vi "Block DMA.vi"() -> ()   [LabVIEW 2016]
uses:
  <vilib>/NI/GE Reflective Memory Driver/Typedefs/GE 5565PIORC.Typedef.DMA Wait Mode.ctl
  <vilib>/NI/GE Reflective Memory Driver/GE 5565PIORC.lvclass/GE 5565PIORC.ctl
  <vilib>/NI/GE Reflective Memory Driver/Methods/GE 5565PIORC.DMA.Block.Write (String).vi
  <vilib>/NI/GE Reflective Memory Driver/Methods/GE 5565PIORC.DMA.Create Transfer (Block).vi
  <vilib>/NI/GE Reflective Memory Driver/Methods/GE 5565PIORC.DMA.Get Transfer Components (Block).vi
  <vilib>/NI/GE Reflective Memory Driver/Methods/GE 5565PIORC.DMA.Block.Read (String).vi
  <vilib>/NI/GE Reflective Memory Driver/Properties/Registers/GE 5565PIORC.Registers.LAS1RR.PCI Address Range.Get.vi
  <vilib>/NI/GE Reflective Memory Driver/Methods/GE 5565PIORC.PXI Interrupts.Enable.vi
  <vilib>/NI/GE Reflective Memory Driver/Properties/Registers/GE 5565PIORC.Registers.DMACSR0.Channel 0 Enable.Set.vi
  <vilib>/NI/GE Reflective Memory Driver/Properties/Registers/GE 5565PIORC.Registers.INTCSR.Local DMA Channel 0 Interrupt Enable.Set.vi
  <vilib>/NI/GE Reflective Memory Driver/Properties/GE 5565PIORC.Read VISA MEMACC.vi
  <vilib>/NI/GE Reflective Memory Driver/Methods/GE 5565PIORC.DMA.Create Transfer (Scatter-Gather).vi
  <vilib>/NI/GE Reflective Memory Driver/Methods/GE 5565PIORC.DMA.Configure.vi
  <vilib>/NI/GE Reflective Memory Driver/Methods/GE 5565PIORC.PXI Interrupts.Discard Events.vi
  <vilib>/NI/GE Reflective Memory Driver/Methods/GE 5565PIORC.DMA.Start.vi
  <vilib>/NI/GE Reflective Memory Driver/Methods/GE 5565PIORC.DMA.Wait for Done.vi
  <vilib>/NI/GE Reflective Memory Driver/Methods/GE 5565PIORC.DMA.Block.Clear.vi
  <vilib>/NI/GE Reflective Memory Driver/Methods/GE 5565PIORC.DMA.Block.Clear (multiple).vi
  <vilib>/NI/GE Reflective Memory Driver/Properties/Registers/GE 5565PIORC.Registers.Local Configuration.Read.vi
  <vilib>/NI/GE Reflective Memory Driver/Properties/Registers/GE 5565PIORC.Registers.Local Configuration.Read (U32).vi
  <vilib>/NI/GE Reflective Memory Driver/Properties/Registers/GE 5565PIORC.Registers.Local Configuration.Read (U8).vi
  <vilib>/NI/GE Reflective Memory Driver/Properties/Registers/GE 5565PIORC.Registers.Local Configuration.Write.vi
  <vilib>/NI/GE Reflective Memory Driver/Properties/Registers/GE 5565PIORC.Registers.Local Configuration.Write (U8).vi
  <vilib>/NI/GE Reflective Memory Driver/Methods/GE 5565PIORC.Bit Manipulation.Set Bit.vi
  <vilib>/NI/GE Reflective Memory Driver/Methods/GE 5565PIORC.Bit Manipulation.Set Bit (U8).vi
  <vilib>/NI/GE Reflective Memory Driver/Properties/Registers/GE 5565PIORC.Registers.Local Configuration.Write (U32).vi
  <vilib>/NI/GE Reflective Memory Driver/Methods/GE 5565PIORC.Bit Manipulation.Set Bit (U32).vi
  <vilib>/NI/GE Reflective Memory Driver/Methods/GE 5565PIORC.DMA.Size.vi
  <vilib>/NI/GE Reflective Memory Driver/Properties/Registers/GE 5565PIORC.Registers.DMADPR0.Direction of Transfer.Set.vi
  <vilib>/NI/GE Reflective Memory Driver/Properties/Registers/GE 5565PIORC.Registers.DMASIZ0.DMA Transfer Size.Set.vi
  <vilib>/NI/GE Reflective Memory Driver/Properties/Registers/GE 5565PIORC.Registers.DMALADR0.Local Address Register.Set.vi
  <vilib>/NI/GE Reflective Memory Driver/Properties/Registers/GE 5565PIORC.Registers.DMAMODE0.Scatter-Gather Mode.Set.vi
  <vilib>/NI/GE Reflective Memory Driver/Properties/Registers/GE 5565PIORC.Registers.DMAPADR0.PCI Address Register.Set.vi
  <vilib>/NI/GE Reflective Memory Driver/Methods/GE 5565PIORC.DMA.Scatter-Gather.Link Block Descriptors.vi
  <vilib>/NI/GE Reflective Memory Driver/Methods/GE 5565PIORC.DMA.Scatter-Gather.Commit Linked Block Descriptors.vi
  <vilib>/NI/GE Reflective Memory Driver/Properties/Registers/GE 5565PIORC.Registers.DMADPR0.Channel 0 First Descriptor Address.Set.vi
  <vilib>/NI/GE Reflective Memory Driver/Methods/GE 5565PIORC.DMA.Get Transfer Components (Scatter-Gather).vi
  <vilib>/Utility/error.llb/Clear Errors.vi
  <vilib>/NI/GE Reflective Memory Driver/Properties/Registers/GE 5565PIORC.Registers.DMACSR0.Channel 0 Start.Set.vi
  <vilib>/NI/GE Reflective Memory Driver/Properties/Registers/GE 5565PIORC.Registers.DMACSR0.Channel 0 Clear Interrupt.Set.vi
  <vilib>/NI/GE Reflective Memory Driver/Methods/GE 5565PIORC.DMA.Poll for Done Signal.vi
  <vilib>/NI/GE Reflective Memory Driver/Methods/GE 5565PIORC.PXI Interrupts.Wait for Event.vi
  <vilib>/NI/GE Reflective Memory Driver/Methods/GE 5565PIORC.DMA.Block.Clear (single).vi
  <vilib>/NI/GE Reflective Memory Driver/Methods/GE 5565PIORC.Registers.Read.vi
  <vilib>/NI/GE Reflective Memory Driver/Methods/GE 5565PIORC.Registers.Read (U32).vi
  <vilib>/NI/GE Reflective Memory Driver/Methods/GE 5565PIORC.Registers.Read (U8).vi
  <vilib>/NI/GE Reflective Memory Driver/Methods/GE 5565PIORC.Registers.Write.vi
  <vilib>/NI/GE Reflective Memory Driver/Methods/GE 5565PIORC.Registers.Write (U8).vi
  <vilib>/NI/GE Reflective Memory Driver/Methods/GE 5565PIORC.Registers.Write (U32).vi
  <vilib>/NI/GE Reflective Memory Driver/Methods/GE 5565PIORC.DMA.Scatter-Gather.Set Descriptor Params.vi
  <vilib>/NI/GE Reflective Memory Driver/Methods/GE 5565PIORC.DMA.Is Done.vi
  <vilib>/NI/GE Reflective Memory Driver/Properties/Registers/GE 5565PIORC.Registers.DMACSR0.Channel 0 Inactive.Get.vi
  <vilib>/NI/GE Reflective Memory Driver/Methods/GE 5565PIORC.Bit Manipulation.Get Bit.vi
  <vilib>/NI/GE Reflective Memory Driver/Methods/GE 5565PIORC.Bit Manipulation.Get Bit (U8).vi
  <vilib>/NI/GE Reflective Memory Driver/Methods/GE 5565PIORC.Round Up to Nearest 8.vi
  <vilib>/NI/GE Reflective Memory Driver/Methods/GE 5565PIORC.Round Up to Nearest 16.vi
  <vilib>/NI/GE Reflective Memory Driver/GE 5565PIORC.lvclass
panel:
  out "Success?":bool
  out "Read Timed Out?":bool
  out "Write Timed Out?":bool
  in  "RFM offset":u32 format="%.0x"
  in  "Transfer Size (bytes)":u32=1024000
  in  "Wait Mode":T1
  in  "VISA Resource Name":refnum<visa-resource-name>="PXI4::14::INSTR"
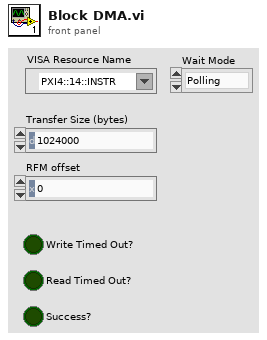
[diagram p1: front panel]
types:
  T1 = typedef "GE 5565PIORC.lvclass/GE 5565PIORC.Typedef.DMA Wait Mode.ctl" = enum16{"Polling", "Interrupt"}
  T2 = typedef "GE 5565PIORC.lvclass/GE 5565PIORC.Typedef.DMA Block Descriptor.ctl" = cluster{"descriptor ptr (VISA)":u32, "descriptor ptr (RFM)":u32, "descriptor size":u32, "descriptor params":T3}
  T3 = typedef "GE 5565PIORC.lvclass/GE 5565PIORC.Typedef.DMA Block Descriptor Params.ctl" = cluster{"data ptr (lower)":u32, "data ptr (upper)":u32, "data size":u32, "next descriptor ptr":u32}
  T4 = typedef "GE 5565PIORC.lvclass/GE 5565PIORC.Typedef.DMA Transfer Spec.ctl" = cluster{"RFM offset":u32, "Block Descriptors":T2[]}
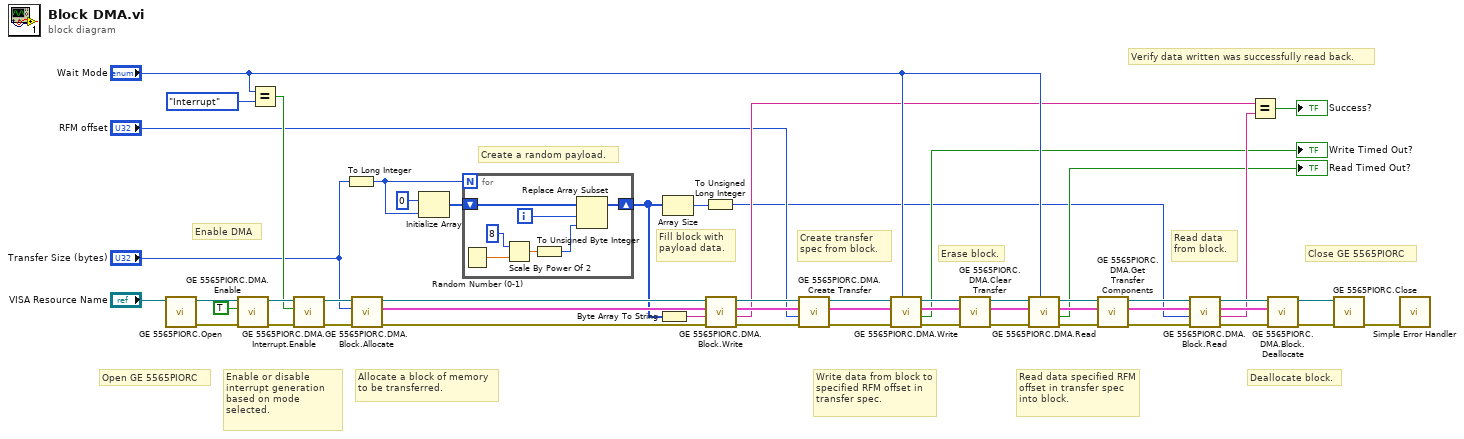
[diagram p0: block diagram]
diagram:
  # "Verify data written was successfully read back."
  # "Close GE 5565PIORC"
  # "Deallocate block."
  # "Erase block."
  # "Read data from block."
  # "Read data specified RFM offset in transfer spec into block."
  # "Write data from block to specified RFM offset in transfer spec."
  # "Create transfer spec from block."
  # "Fill block with payload data."
  # "Allocate a block of memory to be transferred."
  # "Enable or disable interrupt generation based on mode selected."
  # "Enable DMA"
  # "Open GE 5565PIORC"
  # "Create a random payload."
  n1 = call <vilib>:"GE 5565PIORC.Open.vi"("VISA resource name"="VISA Resource Name") -> ("error out"=w50:errorcluster, "GE 5565PIORC"=w51:refnum<class "GE 5565PIORC.lvclass">)  [unwired: 9 in]
  n2 = call <vilib>:"GE 5565PIORC.DMA.Enable.vi"("error in (no error)"=w50, "enable (T)"=TRUE, "GE 5565PIORC in"=w51) -> ("error out"=w48:errorcluster, "GE 5565PIORC out"=w47:refnum<class "GE 5565PIORC.lvclass">)  [unwired: 7 in]
  n3 = Equal?(x="Wait Mode", y=GE_5565PIORC.Typedef.DMA_Wait_Mode."Interrupt") -> (x = y?=w38:bool)
  n4 = call <vilib>:"GE 5565PIORC.DMA.Interrupt.Enable.vi"("error in (no error)"=w48, "enable (T)"=w38, "GE 5565PIORC in"=w47) -> ("error out"=w44:errorcluster, "GE 5565PIORC out"=w45:refnum<class "GE 5565PIORC.lvclass">)  [unwired: 7 in]
  n5 = To Long Integer(number="Transfer Size (bytes)") -> (32bit integer=w32:i32)
  n6 = call <vilib>:"GE 5565PIORC.DMA.Block.Allocate.vi"("error in (no error)"=w44, "size in bytes"="Transfer Size (bytes)", "GE 5565PIORC in"=w45) -> ("error out"=w25:errorcluster, "Block Descriptor"=w22:T2, "GE 5565PIORC out"=w26:refnum<class "GE 5565PIORC.lvclass">)  [unwired: 6 in]
  n7 = Initialize Array(u8 0, w32) -> (w42:u8[])
  n8 = for {
    N: w32 -> [_]
    shift-right: [w58] -> w18
    shift-left: w42 -> [w59]
    i -> [w57]
    n9 = Random Number (0-1)() -> (number: 0 to 1=w56:dbl)
    n10 = Scale By Power Of 2(n=i16 8, x=w56) -> (x*2^n=w54:dbl)
    n11 = To Unsigned Byte Integer(number=w54) -> (unsigned 8bit integer=w53:u8)
    n12 = Replace Array Subset(array=w59, new element=w53, index=w57) -> (w58:u8[])
  }
  n13 = Byte Array To String(unsigned byte array=w18) -> (string=w19:string)
  n14 = Array Size(array=w18) -> (size(s)=w4:i32)
  n15 = To Unsigned Long Integer(number=w4) -> (unsigned 32bit integer=w1:u32)
  n16 = call-poly <vilib>:"GE 5565PIORC.DMA.Block.Write.vi"("error in (no error)"=w25, "data"=w19, "Block Descriptor in"=w22, "GE 5565PIORC in"=w26) -> ("error out"=w23:errorcluster, "data out"=w20:string, "Block Descriptor out"=w21:T2, "GE 5565PIORC out"=w24:refnum<class "GE 5565PIORC.lvclass">)  [unwired: 4 in]
  n17 = call-poly <vilib>:"GE 5565PIORC.DMA.Create Transfer.vi"("error in (no error)"=w23, "RFM offset"="RFM offset", "Block Descriptor"=w21, "GE 5565PIORC in"=w24) -> ("error out"=w39:errorcluster, "DMA Transfer Spec"=w40:T4, "GE 5565PIORC out"=w41:refnum<class "GE 5565PIORC.lvclass">)  [unwired: 4 in, 1 out]
  n18 = call <vilib>:"GE 5565PIORC.DMA.Write.vi"("wait mode (polling)"="Wait Mode", "error in (no error)"=w39, "DMA Transfer Spec"=w40, "GE 5565PIORC in"=w41) -> ("error out"=w16:errorcluster, "timed out?"=→"Write Timed Out?":bool, "DMA Transfer Spec dup"=w15:T4, "GE 5565PIORC out"=w17:refnum<class "GE 5565PIORC.lvclass">)  [unwired: 4 in]
  n19 = call <vilib>:"GE 5565PIORC.DMA.Clear Transfer.vi"("error in (no error)"=w16, "DMA Transfer Spec in"=w15, "GE 5565PIORC in"=w17) -> ("error out"=w13:errorcluster, "DMA Transfer Spec out"=w12:T4, "GE 5565PIORC out"=w14:refnum<class "GE 5565PIORC.lvclass">)  [unwired: 6 in]
  n20 = call <vilib>:"GE 5565PIORC.DMA.Read.vi"("wait mode (polling)"="Wait Mode", "error in (no error)"=w13, "DMA Transfer Spec"=w12, "GE 5565PIORC in"=w14) -> ("error out"=w9:errorcluster, "timed out?"=→"Read Timed Out?":bool, "DMA Transfer Spec dup"=w8:T4, "GE 5565PIORC out"=w10:refnum<class "GE 5565PIORC.lvclass">)  [unwired: 4 in]
  n21 = call-poly <vilib>:"GE 5565PIORC.DMA.Get Transfer Components.vi"("error in (no error)"=w9, "DMA Transfer Spec in"=w8, "GE 5565PIORC in"=w10) -> ("error out"=w5:errorcluster, "Block Descriptor"=w6:T2, "GE 5565PIORC out"=w7:refnum<class "GE 5565PIORC.lvclass">)  [unwired: 5 in, 1 out]
  n22 = call-poly <vilib>:"GE 5565PIORC.DMA.Block.Read.vi"("error in (no error)"=w5, "bytes to read"=w1, "Block Descriptor in"=w6, "GE 5565PIORC in"=w7) -> ("error out"=w29:errorcluster, "data"=w27:string, "Block Descriptor out"=w28:T2, "GE 5565PIORC out"=w30:refnum<class "GE 5565PIORC.lvclass">)  [unwired: 4 in]
  n23 = Equal?(x=w20, y=w27) -> (x = y?=→"Success?":bool)
  n24 = call <vilib>:"GE 5565PIORC.DMA.Block.Deallocate.vi"("error in (no error)"=w29, "Block Descriptor"=w28, "GE 5565PIORC in"=w30) -> ("error out"=w35:errorcluster, "GE 5565PIORC out"=w36:refnum<class "GE 5565PIORC.lvclass">)  [unwired: 7 in]
  n25 = call <vilib>:"GE 5565PIORC.Close.vi"("error in (no error)"=w35, "GE 5565PIORC in"=w36) -> ("error out"=w34:errorcluster)  [unwired: 8 in, 1 out]
  n26 = call <vilib>:"Simple Error Handler.vi"("error in (no error)"=w34) -> ()  [unwired: 4 in, 5 out]
